vi "doTestingLab.vi"() -> ()   [LabVIEW 2009, in "run.lvlib"]
uses:
  run.lvlib
  Channels/Digital/DigitalOutput.lvclass
  Channels/VoltOutput/AnalogOutput.lvclass
  SingleAtoms/DGImagingController/DGImagingController.lvclass
panel:
  out "data":T1 {"Timestamps ms" format="%#.6g"}
  out "appended array":dbl[][](array[numeric])
  in  "Data":T2={"Timestamps ms"=[0.0, 2000.0, 2000.2, 3000.0, 4000.0, 5000.0], "Camera"=[[1, 0], [1, 1], [0, 0], [0, 0], [1, 0], [0, 0]], "AnalogData"=[[1, 0, 0, 1], [1, 1, 0, 1], [1, 1, 0, 0], [1, 1, 0, 0], [1, 1, 0, 0], [1, 0, 0, 0]], "Coils Volts"=2.2, "Shutter Volts"=2.0, "AOM2 Volts"=0.3, "Array"=[-0.1, 0.336, 0.336, 0.336, -0.1, -0.1]} {"AnalogData" items=["On"=1, "Off"=0]; "Camera" items=["On"=1, "Off"=0, "Init"=2]; "Timestamps ms" format="%#_10g"}
  in  "stop":bool
  # "Stop Acquisition Before\nis finished."
  # "Analog Output Channels"
  # "Digital Port0"
  # "Line P0.1"
  # "Line P0.2"
  # "Line P0.3"
  # "Detuning"
  # "Camera"
  # "Imaging"
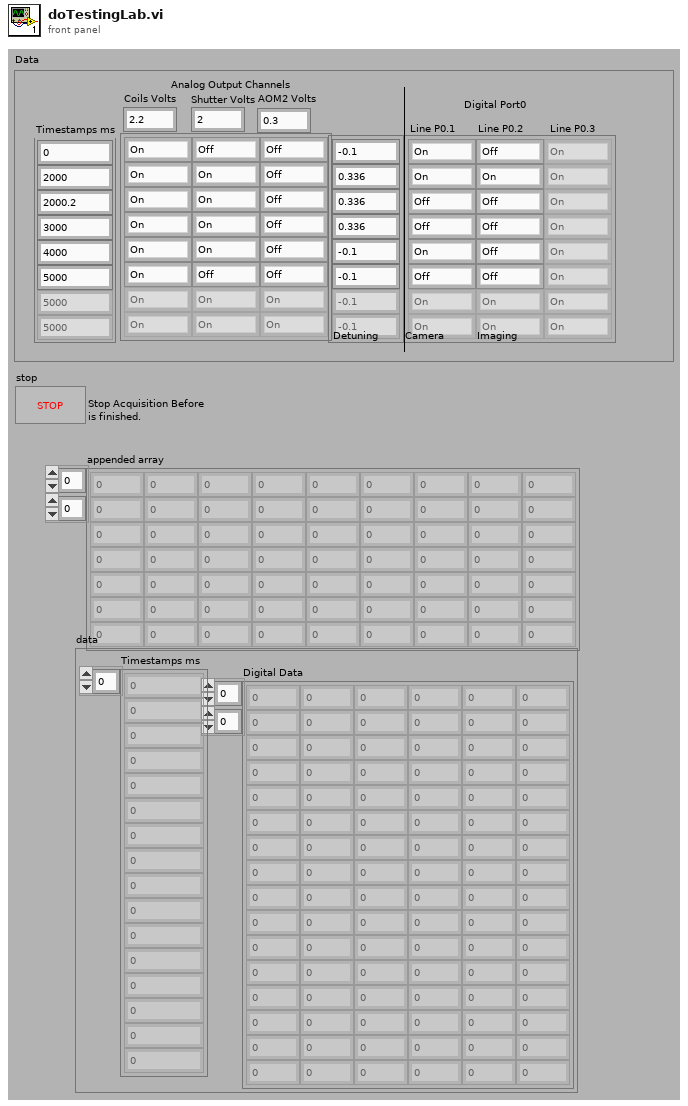
[diagram p1: front panel]
types:
  T1 = cluster{"Timestamps ms":dbl[], "Digital Data":dbl[][]}
  T2 = cluster{"Timestamps ms":dbl[], "Camera":u16[][], "AnalogData":u16[][], "Coils Volts":dbl, "Shutter Volts":dbl, "AOM2 Volts":dbl, "Array":dbl[]}
  T3 = cluster{"Name":string, "Channels":string, "Ranges":dbl[]}
  T4 = cluster{"Master Clock source":string, "Master Clock rate":dbl, "Start trigger line":string, "Scan rate":dbl, "Stop trigger line":string, dbl}
  T5 = cluster{"Clock source":string, "Clock rate":dbl, "Start trigger line":string, "Sample Rate":dbl, dbl}
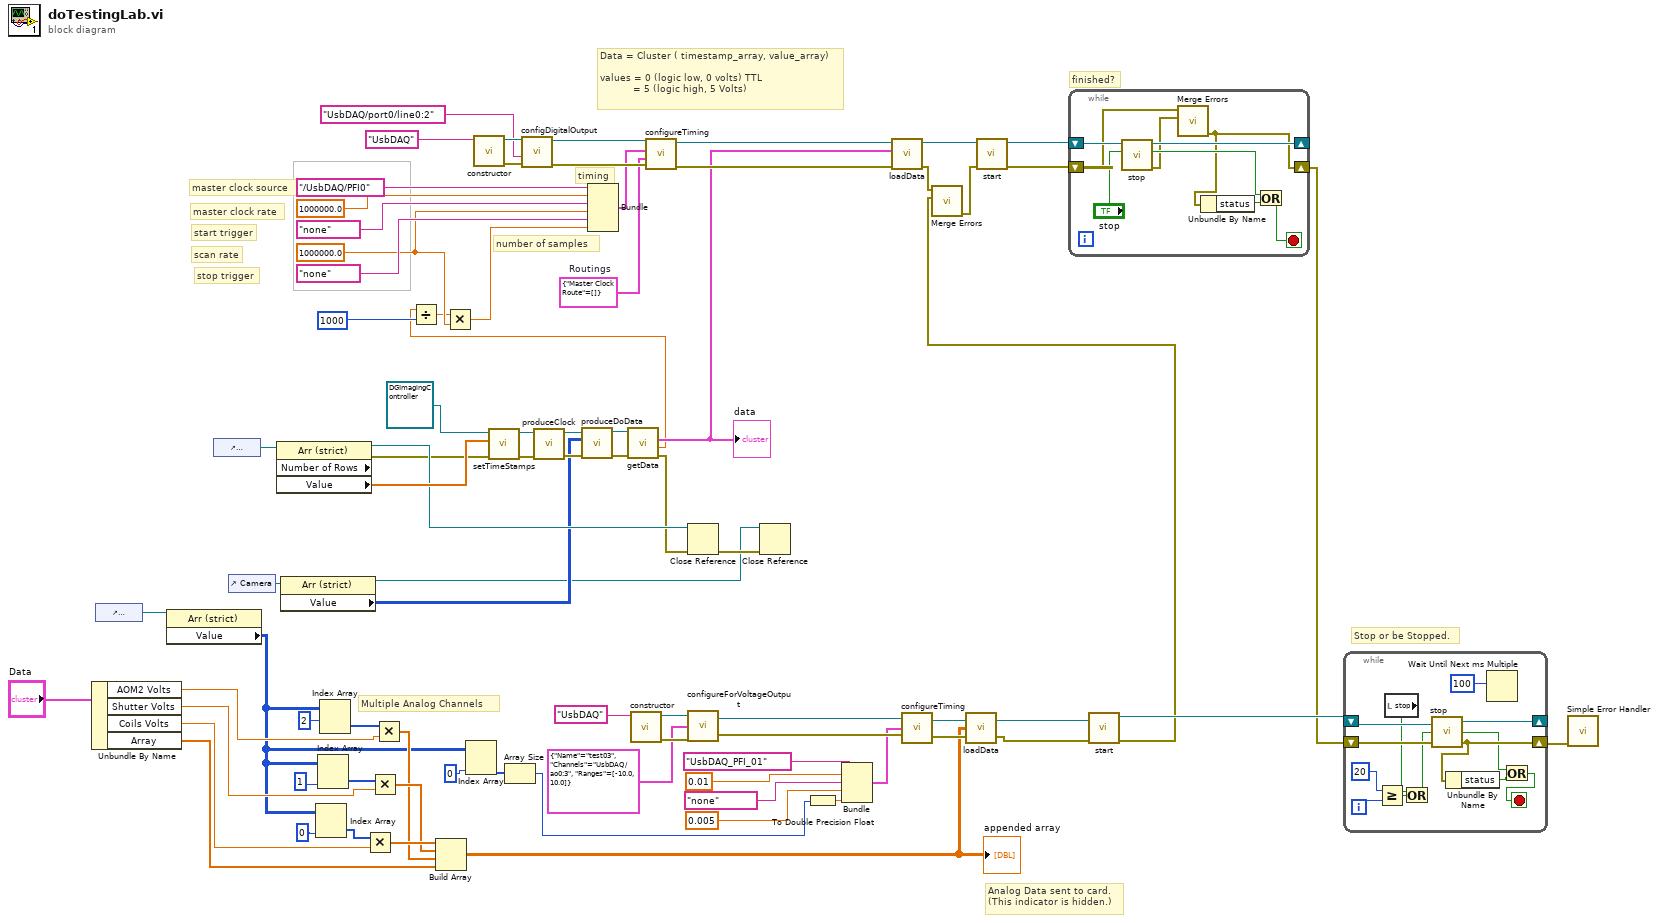
[diagram p0: block diagram]
diagram:
  w70 = cluster{"Master Clock Route":string[]} {"Master Clock Route"=[]}  # Routings
  w64 = 1000000.0 ("Scan rate")
  # "Analog Data sent to card.\n(This indicator is hidden.)"
  # "Multiple Analog Channels"
  # "Stop or be Stopped."
  # "Data = Cluster ( timestamp_array, value_array)\n\nvalues = 0 (logic low, 0 volts) TTL\n           = 5 (logic high, 5 Volts)"
  # "master clock source"
  # "number of samples"
  # "stop trigger"
  # "scan rate"
  # "start trigger"
  # "master clock rate"
  # "finished?"
  # "timing"
  n1 = Unbundle By Name("Data") -> ("AOM2 Volts"=w27:dbl, "Shutter Volts"=w26:dbl, "Coils Volts"=w25:dbl, "Array"=w19:dbl[])
  n2 = control-ref of="AnalogData"() -> (w20:refnum<vi>)
  n3 = property class="Arr (strict)"(reference=w20) -> ("Value"=w23:u16[][])  [unwired: 1 in, 2 out]
  n4 = control-ref of="Timestamps ms"() -> (w38:refnum<vi>)
  n5 = control-ref of="Camera"() -> (w37:refnum<vi>)
  n6 = property class="Arr (strict)" props=["Number of Rows", "Value"](reference=w38) -> (reference out=w7:refnum<vi>, error out=w3:errorcluster, "Value"=w8:dbl[])  [unwired: 1 in, 1 out]
  n7 = property class="Arr (strict)"(reference=w37) -> (reference out=w5:refnum<vi>, "Value"=w6:u16[][])  [unwired: 1 in, 1 out]
  n8 = Index Array(array=w23, index (col)=0) -> (element=w28:u16[])  [unwired: 1 in]
  n9 = Index Array(array=w23, index (col)=1) -> (element=w33:u16[])  [unwired: 1 in]
  n10 = Index Array(array=w23, index (col)=2) -> (element=w31:u16[])  [unwired: 1 in]
  n11 = Multiply(x=w28, y=w25) -> (x*y=w35:dbl[])
  n12 = Multiply(x=w33, y=w26) -> (x*y=w30:dbl[])
  n13 = Multiply(x=w31, y=w27) -> (x*y=w29:dbl[])
  n14 = Build Array(w35, w30, w29, w19) -> (w18:dbl[][])
  "appended array" <- w18
  n15 = Index Array(array=w23, index (col)=0) -> (element=w24:u16[])  [unwired: 1 in]
  n16 = call "constructor.vi"("deviceName"="UsbDAQ") -> ("error out"=w67:errorcluster, "DigitalOutput out"=w68:refnum<class "DigitalOutput.lvclass">)  [unwired: 9 in]
  n17 = call "setTimeStamps.vi"("error in (no error)"=w3, "Timestamps ms"=w8, "DGImagingController.lvclass in"=refnum<class "DGImagingController.lvclass"> refnum ("SingleAtoms.lvlib:DGImagingController.lvclass")) -> ("error out"=w15:errorcluster, "DGImagingController.lvclass out"=w16:refnum<class "DGImagingController.lvclass">)  [unwired: 7 in]
  n18 = Array Size(array=w24) -> (size(s)=w17:i32)
  n19 = call-dynamic "configDigitalOutput.vi"("error in (no error)"=w67, "Physical Channels"="UsbDAQ/port0/line0:2", "DigitalOutput in"=w68) -> ("error out"=w80:errorcluster, "DigitalOutput out"=w81:refnum<class "DigitalOutput.lvclass">)  [unwired: 7 in]
  n20 = call "produceClock.vi"("error in (no error)"=w15, "DGImagingController in"=w16) -> ("error out"=w13:errorcluster, "DGImagingController out"=w14:refnum<class "DGImagingController.lvclass">)  [unwired: 8 in]
  n21 = call "produceDoData.vi"("error in (no error)"=w13, "Digital Data"=w6, "DGImagingController in"=w14) -> ("error out"=w12:errorcluster, "DGImagingController out"=w11:refnum<class "DGImagingController.lvclass">)  [unwired: 7 in]
  n22 = call "getData.vi"("error in (no error)"=w12, "DGImagingController in"=w11) -> ("error out"=w4:errorcluster, "last timeStamp"=w1:dbl, "data"=w2:T1)  [unwired: 6 in, 1 out]
  "data" <- w2
  n23 = Divide(x=w1, y=1000) -> (x/y=w63:dbl)
  n24 = Multiply(x=w63, y=w64) -> (x*y=w56:dbl)
  n25 = Bundle("Master Clock source"="/UsbDAQ/PFI0", "Master Clock rate"=1000000.0, "Start trigger line"="none", "Scan rate"=w64, "Stop trigger line"="none", w56) -> (w71:T4)  [unwired: 1 in]
  n26 = call "constructor.vi"("deviceName"="UsbDAQ") -> ("error out"=w48:errorcluster, "AnalogOutput out"=w49:refnum<class "AnalogOutput.lvclass">)  [unwired: 9 in]
  n27 = call-dynamic "configureTiming.vi"("error in (no error)"=w80, "Routings"=w70, "Timing"=w71, "DigitalOutput in"=w81) -> ("error out"=w78:errorcluster, "DigitalOutput out"=w79:refnum<class "DigitalOutput.lvclass">)  [unwired: 6 in]
  n28 = Close Reference(reference=w7, error in (no error)=w4) -> (error out=w9:errorcluster)
  n29 = call-dynamic "configureForVoltageOutput.vi"("error in (no error)"=w48, "Output Properties"=T3 {"Name"="test03", "Channels"="UsbDAQ/ao0:3", "Ranges"=[-10.0, 10.0]}, "AnalogOutput in"=w49) -> ("error out"=w54:errorcluster, "AnalogOutput out"=w55:refnum<class "AnalogOutput.lvclass">)
  n30 = Close Reference(reference=w5, error in (no error)=w9) -> ()  [unwired: 1 out]
  n31 = To Double Precision Float(number=w17) -> (double precision float=w40:dbl)
  n32 = Bundle("Clock source"="UsbDAQ_PFI_01", "Clock rate"=0.01, "Start trigger line"="none", "Sample Rate"=0.005, w40) -> (w45:T5)  [unwired: 1 in]
  n33 = call-dynamic "loadData.vi"("error in (no error)"=w78, "Data"=w2, "DigitalOutput in"=w79) -> ("error out"=w60:errorcluster, "DigitalOutput out"=w77:refnum<class "DigitalOutput.lvclass">)  [unwired: 7 in]
  n34 = call-dynamic "configureTiming.vi"("error in (no error)"=w54, "Timing"=w45, "AnalogOutput in"=w55) -> ("error out"=w52:errorcluster, "AnalogOutput out"=w53:refnum<class "AnalogOutput.lvclass">)
  n35 = call-dynamic "loadData.vi"("error in (no error)"=w52, "Data"=w18, "AnalogOutput in"=w53) -> ("error out"=w50:errorcluster, "AnalogOutput out"=w51:refnum<class "AnalogOutput.lvclass">)
  n36 = call-dynamic "start.vi"("error in (no error)"=w50, "AnalogOutput in"=w51) -> ("error out"=w58:errorcluster, "AnalogOutput out"=w61:refnum<class "AnalogOutput.lvclass">)  [unwired: 8 in]
  n37 = call <vilib>:"Merge Errors.vi"("error in 2 (no error)"=w58, "error in 1 (no error)"=w60) -> ("error out"=w59:errorcluster)  [unwired: 5 in]
  n38 = call-dynamic "start.vi"("error in (no error)"=w59, "DigitalOutput in"=w77) -> ("error out"=w69:errorcluster, "DigitalOutput out"=w76:refnum<class "DigitalOutput.lvclass">)  [unwired: 8 in]
  n39 = while {
    shift-right: [w89] -> _
    shift-left: w76 -> [w90]
    shift-right: [w82] -> w57
    shift-left: w69 -> [w84]
    stop <- w86 stop-if-true
    n40 = call-dynamic "stop.vi"("stop"="stop", "DigitalOutput in"=w90) -> ("error out"=w83:errorcluster, "stopped"=w88:bool, "DigitalOutput out"=w89:refnum<class "DigitalOutput.lvclass">)  [unwired: 7 in]
    n41 = call <vilib>:"Merge Errors.vi"("error in 2 (no error)"=w83, "error in 1 (no error)"=w84) -> ("error out"=w82:errorcluster)  [unwired: 5 in]
    n42 = Unbundle By Name(w82) -> ("status"=w87:bool)
    n43 = Or(x=w88, y=w87) -> (x .or. y?=w86:bool)
  }
  n44 = while {
    shift-right: [w101] -> _
    shift-left: w61 -> [w102]
    shift-right: [w100] -> w39
    shift-left: w57 -> [w103]
    i -> [w95]
    stop <- w98 stop-if-true
    n45 = Greater Or Equal?(x=20, y=w95) -> (x >= y?=w94:bool)
    n46 = local read "stop"() -> (w92:bool)
    n47 = Or(x=w92, y=w94) -> (x .or. y?=w91:bool)
    n48 = call-dynamic "stop.vi"("error in (no error)"=w103, "stop"=w91, "AnalogOutput in"=w102) -> ("error out"=w100:errorcluster, "Stopped"=w99:bool, "AnalogOutput out"=w101:refnum<class "AnalogOutput.lvclass">)
    n49 = Unbundle By Name(w100) -> ("status"=w93:bool)
    n50 = Wait Until Next ms Multiple(millisecond multiple=100) -> ()  [unwired: 1 out]
    n51 = Or(x=w99, y=w93) -> (x .or. y?=w98:bool)
  }
  n52 = call <vilib>:"Simple Error Handler.vi"("error in (no error)"=w39) -> ()  [unwired: 4 in, 5 out]
